vi "ROI_Overlay.vi"(10 "XYZ":T1, 11 "Image In":T2) -> (3 "Image out":T2)   [LabVIEW 2020]
uses:
  <vilib>/vision/Image Controls.llb/IMAQ Image.ctl
  ROIDataControl.ctl
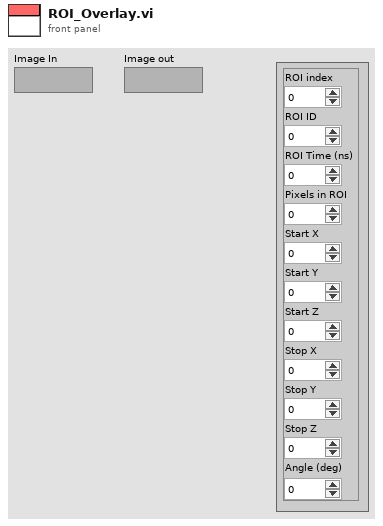
[diagram p1: front panel]
types:
  T1 = typedef "ROIDataControl.ctl" = cluster{"ROI index":i16, "ROI ID":i16, "ROI Time (ns)":sgl, "Pixels in ROI":i16, "Start X":dbl, "Start Y":dbl, "Start Z":dbl, "Stop X":dbl, "Stop Y":dbl, "Stop Z":i16, "Angle (deg)":dbl}
  T2 = typedef "IMAQ Image.ctl" = refnum<image>
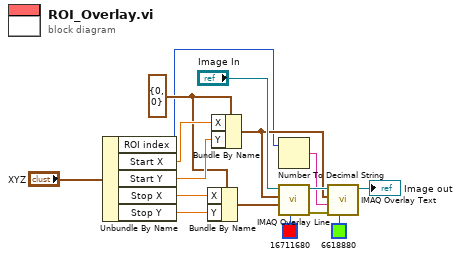
[diagram p0: block diagram]
diagram:
  w11 = cluster{"X":i32, "Y":i32} {"X"=0, "Y"=0} ("Start Point")
  n1 = Unbundle By Name("XYZ") -> ("ROI index"=w2:i16, "Start X"=w13:dbl, "Start Y"=w12:dbl, "Stop X"=w10:dbl, "Stop Y"=w9:dbl)
  n2 = Bundle By Name(cluster=w11, "X"=w10, "Y"=w9) -> (w8:cluster{"X":i32, "Y":i32})
  n3 = Bundle By Name(cluster=w11, "X"=w13, "Y"=w12) -> (w5:cluster{"X":i32, "Y":i32})
  n4 = Number To Decimal String(number=w2) -> (decimal integer string=w1:string)  [unwired: 1 in]
  n5 = call "IMAQ Overlay Line"("Color"=u32 16711680, "End Point"=w8, "Start Point"=w5, "Image"="Image In") -> ("error out"=w3:errorcluster, "Image Out"=w7:T2)  [unwired: 6 in]
  n6 = call "IMAQ Overlay Text"("Text Color (black)"=u32 6618880, "error in (no error)"=w3, "String"=w1, "Origin"=w5, "Image"=w7) -> ("Image Out"=→"Image out":T2)  [unwired: 5 in, 1 out]
